vi "CuffGraspButtons.vi"(0 "error in":errorcluster, 2 "Cuff Inputs":T2={"Side"=enum."left", "Button"=enum."cuff", "Position"=enum."lower"}, 3 "node":string) -> (1 "error out":errorcluster, 4 "Digital IO State":cluster{"state":i8, "is input only":bool})   [LabVIEW 2012]
doc: "Reads the state of the cuff grasp buttons"
uses:
  <userlib>/ROS for LabVIEW Software/ROS/Code/SubVIs/BaxterSide.ctl
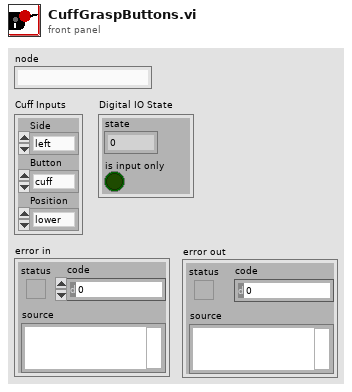
[diagram p1: front panel]
types:
  T1 = typedef "BaxterSide.ctl" = enum16{"left", "right"}
  T2 = cluster{"Side":T1, "Button":enum16{"button", "cuff"}, "Position":enum16{"upper", "lower", "shoulder"}}
  T3 = enum16{"left_lower_cuff", "right_lower_cuff", "left_lower_button", "right_lower_button", "left_upper_button", "right_upper_button", "left_shoulder_button", "right_shoulder_button"}
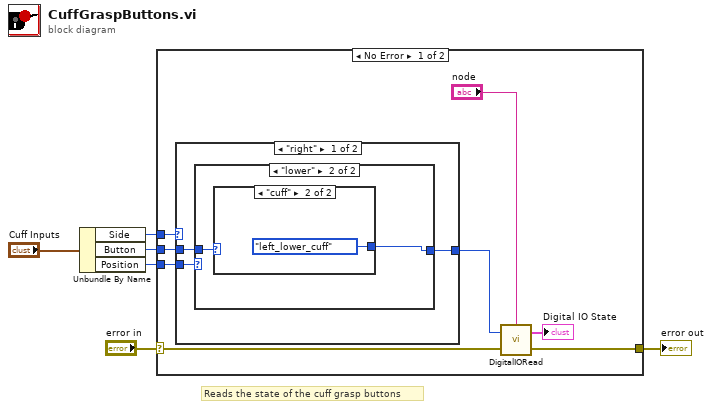
[diagram p0: block diagram]
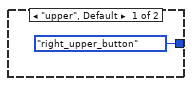
[diagram p2: hidden frame]
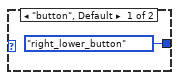
[diagram p3: hidden frame]
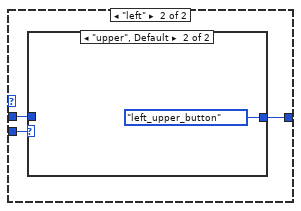
[diagram p4: hidden frame]
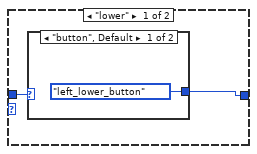
[diagram p5: hidden frame]
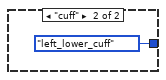
[diagram p6: hidden frame]
diagram:
  # "Reads the state of the cuff grasp buttons"
  n1 = Unbundle By Name("Cuff Inputs") -> ("Side"=w3:T1, "Button"=w1:enum16{"button", "cuff"}, "Position"=w2:enum16{"upper", "lower", "shoulder"})
  n2 = case shown="No Error" "error in" {
    selector: "error in" -> [w8 w31]
    tunnel: [w14 w31] -> w6
    tunnel: w3 -> [w12 _]
    tunnel: w2 -> [w9 _]
    tunnel: w1 -> [w7 _]
    frame No Error {
      n3 = case shown="\"right\"" w12 {
        tunnel: [w17 w25] -> w11
        tunnel: w9 -> [w16 w24]
        tunnel: w7 -> [w15 w23]
        frame "right" {
          n4 = case shown="\"lower\"" w16 {
            tunnel: [T3."right_upper_button" ("Component") w20] -> w17
            tunnel: w15 -> [_ w19]
            frame "upper", Default {
            }
            frame "lower" {
              n5 = case shown="\"cuff\"" w19 {
                tunnel: [T3."right_lower_button" ("Component") T3."left_lower_cuff" ("Component")] -> w20
                frame "button", Default {
                }
                frame "cuff" {
                }
              }
            }
          }
        }
        frame "left" {
          n6 = case shown="\"upper\", Default" w24 {
            tunnel: [w27 T3."left_upper_button" ("Component")] -> w25
            tunnel: w23 -> [w26 _]
            frame "lower" {
              n7 = case shown="\"button\", Default" w26 {
                tunnel: [T3."left_lower_button" ("Component") T3."left_lower_cuff" ("Component")] -> w27
                frame "button", Default {
                }
                frame "cuff" {
                }
              }
            }
            frame "upper", Default {
            }
          }
        }
      }
      n8 = call <userlib>:"DigitalIORead.vi"("error in"=w8, "Component"=w11, "node"="node") -> ("error out"=w14:errorcluster, "Digital IO State"=→"Digital IO State":cluster{"state":i8, "is input only":bool})
    }
    frame Error {
    }
  }
  "error out" <- w6
